vi "tearDown.vi"(8 "error in (no error)":errorcluster, 11 "reference in":refnum<class "SLSC 12201 System Tests.lvclass">) -> (0 "error out":errorcluster, 3 "reference out":refnum<class "SLSC 12201 System Tests.lvclass">)   [LabVIEW 2015, in "SLSC 12201 System Tests.lvclass"]
doc: "tearDown runs after the test method has completed. Use this method to clean up any operations or references that were opened by setUp or the test method. Unit tests should be independent of other unit tests so this VI should ensure that the next test can run in a 'clean' test environment."
uses:
  SLSC 12201 System Tests.lvclass
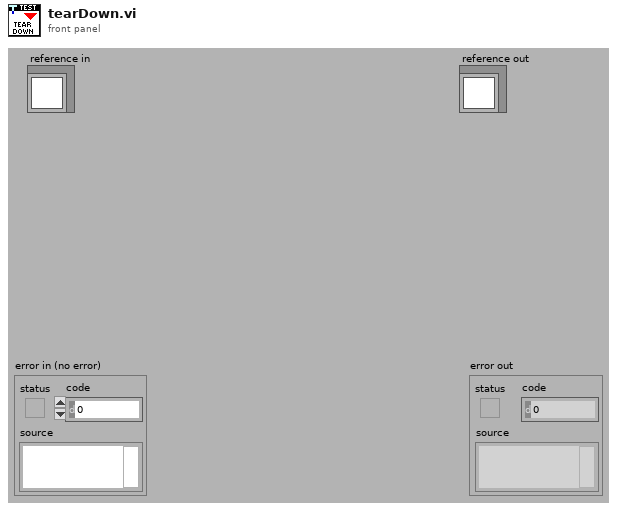
[diagram p1: front panel]
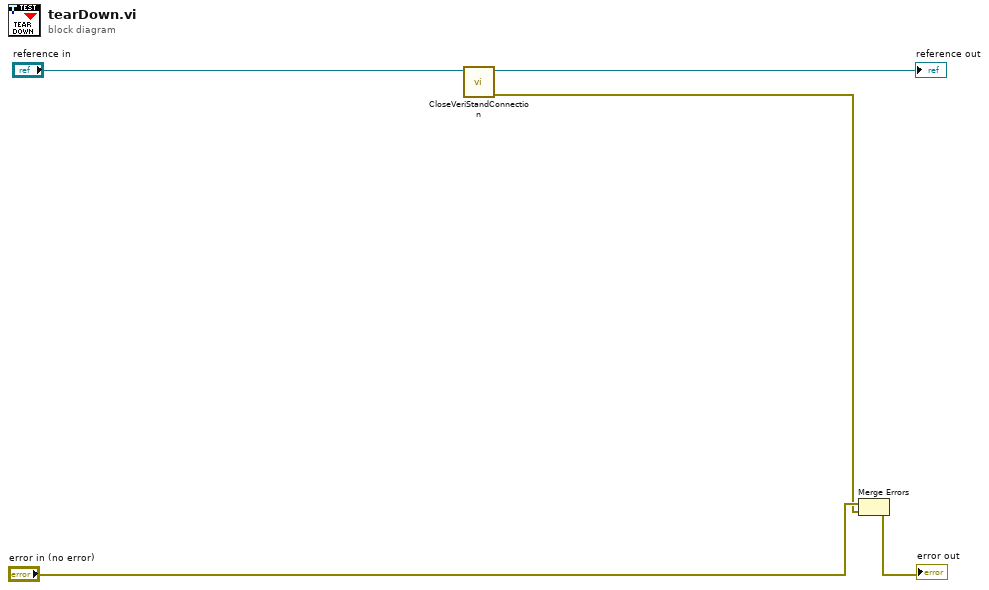
[diagram p0: block diagram]
diagram:
  n1 = call-dynamic "CloseVeriStandConnection.vi"("VeriStand Test Case in"="reference in") -> ("error out"=w1:errorcluster, "VeriStand Test Case out"=→"reference out":refnum<class "SLSC 12201 System Tests.lvclass">)  [unwired: 9 in]
  n2 = Merge Errors("error in (no error)", w1) -> (→"error out":errorcluster)
